vi "Read Stop checjking if OK.vi"(8 "error in (no error)":errorcluster, 11 "Get OSF Status Msg in":refnum<class "Get OSF Status Msg.lvclass">) -> (0 "error out":errorcluster, 2 "Stop checjking if OK":bool, 3 "Get OSF Status Msg out":refnum<class "Get OSF Status Msg.lvclass">)   [LabVIEW 2020, in "Get OSF Status Msg.lvclass"]
uses:
  Get OSF Status Msg.lvclass
  Get OSF Status Msg.lvclass/Get OSF Status Msg.ctl
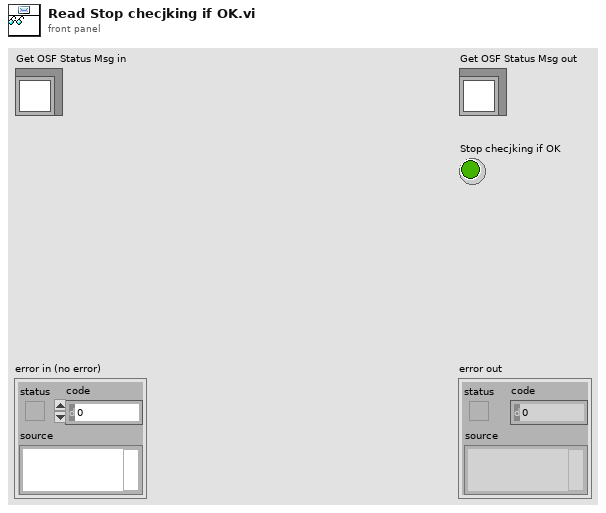
[diagram p1: front panel]
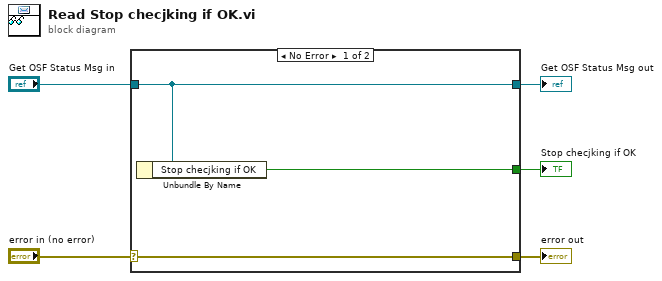
[diagram p0: block diagram]
diagram:
  n1 = case shown="No Error" "error in (no error)" {
    selector: "error in (no error)" -> [w8 w9]
    tunnel: [w8 w9] -> w4
    tunnel: [w7 w10] -> w2
    tunnel: "Get OSF Status Msg in" -> [w7 w10]
    tunnel: [w6 _] -> w1
    frame No Error {
      n2 = Unbundle By Name(w7) -> ("Stop checjking if OK"=w6:bool)
    }
    frame Error {
    }
  }
  "error out" <- w4
  "Get OSF Status Msg out" <- w2
  "Stop checjking if OK" <- w1
